vi "Split Image Array.vi"(6 "Limit":u8=100, 8 "Error In":errorcluster, 11 "Image (U8)":u8[][](array[numeric])) -> (0 "error out":errorcluster, 2 "Image Lower":bool[][](array[boolean]), 3 "Image Upper":bool[][](array[boolean]))   [LabVIEW 2015]
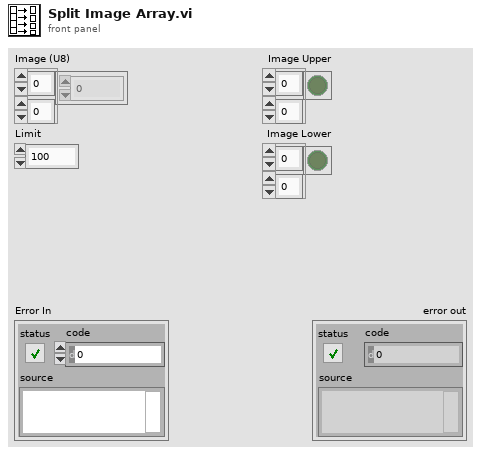
[diagram p1: front panel]
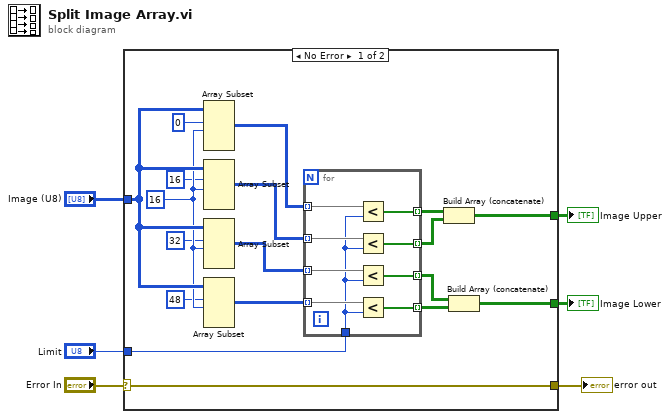
[diagram p0: block diagram]
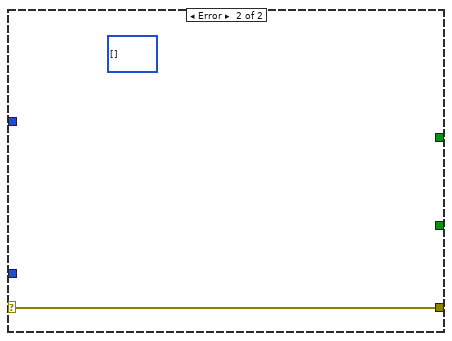
[diagram p2: hidden frame]
diagram:
  n1 = case shown="No Error" "Error In" {
    selector: "Error In" -> [w18 w34]
    tunnel: "Image (U8)" -> [w24 _]
    tunnel: [w18 w34] -> w4
    tunnel: "Limit" -> [w13 _]
    tunnel: [w8 _] -> w2
    tunnel: [w7 _] -> w1
    frame No Error {
      w23 = 16 ("length")
      n2 = Array Subset(array=w24, index (row)=0 ("index"), length (row)=w23) -> (w17:u8[][])  [unwired: 2 in]
      n3 = Array Subset(array=w24, index (row)=16 ("index"), length (row)=w23) -> (w16:u8[][])  [unwired: 2 in]
      n4 = Array Subset(array=w24, index (row)=32 ("index"), length (row)=w23) -> (w15:u8[][])  [unwired: 2 in]
      n5 = Array Subset(array=w24, index (row)=48 ("index"), length (row)=w23) -> (w14:u8[][])  [unwired: 2 in]
      n6 = for {
        tunnel: w17 -> [w30] mode=indexing
        tunnel: w16 -> [w33] mode=indexing
        tunnel: w15 -> [w32] mode=indexing
        tunnel: w14 -> [w31] mode=indexing
        tunnel: [w29] -> w12 mode=indexing
        tunnel: [w28] -> w11 mode=indexing
        tunnel: [w27] -> w9 mode=indexing
        tunnel: [w26] -> w10 mode=indexing
        tunnel: w13 -> [w25]
        n7 = Less?(x=w30, y=w25) -> (x < y?=w29:bool[])
        n8 = Less?(x=w33, y=w25) -> (x < y?=w28:bool[])
        n9 = Less?(x=w32, y=w25) -> (x < y?=w27:bool[])
        n10 = Less?(x=w31, y=w25) -> (x < y?=w26:bool[])
      }
      n11 = Build Array (concatenate)(w12, w11) -> (w8:bool[][])
      n12 = Build Array (concatenate)(w9, w10) -> (w7:bool[][])
    }
    frame Error {
      (unwired) u8[][] []
    }
  }
  "error out" <- w4
  "Image Upper" <- w2
  "Image Lower" <- w1
